vi "Cell label  alphabetical check.vi"(1 "Cell label 2":string="\nPablo1", 2 "Cell label 1":string="Pablo") -> (0 "Is cell label 1 lower than cell label 2?":bool)   [LabVIEW 2011]
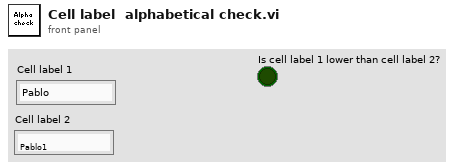
[diagram p1: front panel]
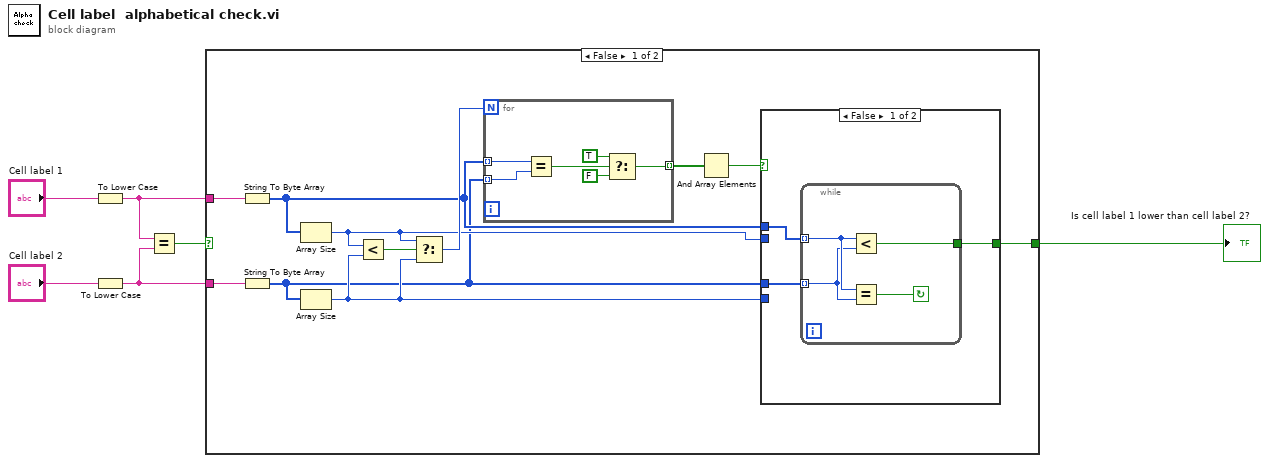
[diagram p0: block diagram]
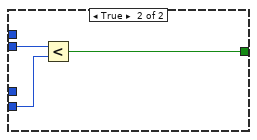
[diagram p2: hidden frame]
diagram:
  n1 = To Lower Case(string="Cell label 1") -> (all lower case string=w6:string)
  n2 = To Lower Case(string="Cell label 2") -> (all lower case string=w5:string)
  n3 = Equal?(x=w6, y=w5) -> (x = y?=w4:bool)
  n4 = case shown="False" w4 {
    selector: w4 -> [_ w34]
    tunnel: w6 -> [w13 _]
    tunnel: w5 -> [w12 _]
    tunnel: [w11 w34] -> w1
    frame False {
      n5 = String To Byte Array(string=w13) -> (unsigned byte array=w8:u8[])
      n6 = String To Byte Array(string=w12) -> (unsigned byte array=w7:u8[])
      n7 = Array Size(array=w8) -> (size(s)=w10:i32)
      n8 = Array Size(array=w7) -> (size(s)=w9:i32)
      n9 = Less?(x=w10, y=w9) -> (x < y?=w17:bool)
      n10 = Select(t=w10, s=w17, f=w9) -> (s? t:f=w16:i32)
      n11 = for {
        N: w16 -> [_]
        tunnel: w8 -> [w33] mode=indexing
        tunnel: w7 -> [w32] mode=indexing
        tunnel: [w28] -> w15 mode=indexing
        n12 = Equal?(x=w33, y=w32) -> (x = y?=w31:bool)
        n13 = Select(t=TRUE ("x < y?"), s=w31, f=FALSE ("x < y?")) -> (s? t:f=w28:bool)
      }
      n14 = And Array Elements(Boolean array=w15) -> (logical AND=w14:bool)
      n15 = case shown="False" w14 {
        tunnel: [w18 w25] -> w11
        tunnel: w10 -> [_ w27]
        tunnel: w9 -> [_ w26]
        tunnel: w8 -> [w19 _]
        tunnel: w7 -> [w20 _]
        frame False {
          n16 = while {
            tunnel: w20 -> [w22] mode=indexing
            tunnel: w19 -> [w23] mode=indexing
            tunnel: [w21] -> w18
            stop <- w24 continue-if-true
            n17 = Less?(x=w23, y=w22) -> (x < y?=w21:bool)
            n18 = Equal?(x=w23, y=w22) -> (x = y?=w24:bool)
          }
        }
        frame True {
          n19 = Less?(x=w27, y=w26) -> (x < y?=w25:bool)
        }
      }
    }
    frame True {
    }
  }
  "Is cell label 1 lower than cell label 2?" <- w1
